vi "HEWH Trim Time.vi"(6 "Data After?":bool, 7 "Max Time":dbl=3606.0 format="%#_13g", 8 "error in (no error)":errorcluster, 11 "FHD-After 1 hour":dbl[][](array[numeric])) -> (0 "error out":errorcluster, 3 "FHD-After 1 hour - Parsed":dbl[][](array[numeric]))   [LabVIEW 2023]
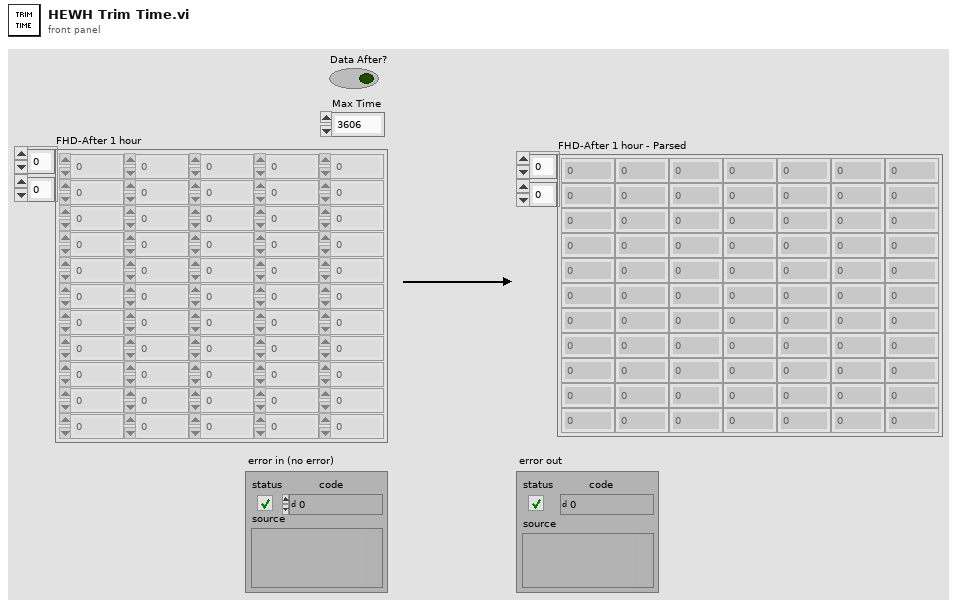
[diagram p1: front panel]
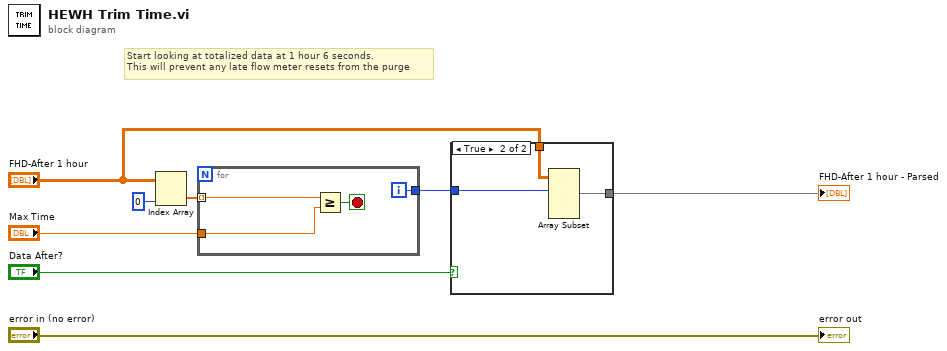
[diagram p0: block diagram]
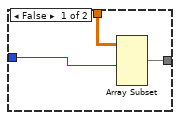
[diagram p2: hidden frame]
diagram:
  # "Start looking at totalized data at 1 hour 6 seconds. \nThis will prevent any late flow meter resets from the purge"
  n1 = Index Array(array="FHD-After 1 hour", index (col)=0 ("disabled index (col)")) -> (element=w7:dbl[])  [unwired: 1 in]
  n2 = for {
    tunnel: w7 -> [w12] mode=indexing
    tunnel: [w10] -> w5
    tunnel: "Max Time" -> [w9]
    i -> [w10]
    stop <- w11 stop-if-true
    n3 = Greater Or Equal?(x=w12, y=w9) -> (x >= y?=w11:bool)
  }
  n4 = case shown="True" "Data After?" {
    tunnel: w5 -> [w14 w18]
    tunnel: "FHD-After 1 hour" -> [w15 w17]
    tunnel: [w13 w16] -> w2
    frame False {
      n5 = Array Subset(array=w15, length (row)=w14) -> (w13:dbl[][])  [unwired: 3 in]
    }
    frame True {
      n6 = Array Subset(array=w17, index (row)=w18) -> (w16:dbl[][])  [unwired: 3 in]
    }
  }
  "FHD-After 1 hour - Parsed" <- w2
  "error out" <- "error in (no error)"
